vi "Create.vi"() -> (0 "error out":errorcluster, 2 "Self Event":refnum<data-value>)   [LabVIEW 2021, in "jettl.lvlib" / "Self Event.lvlib"]
uses:
  Self Event.lvlib
  Msg Strategy/Msg Strategy.lvclass
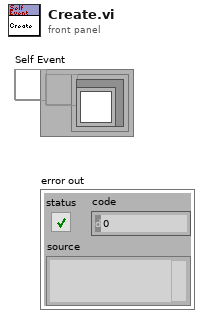
[diagram p1: front panel]
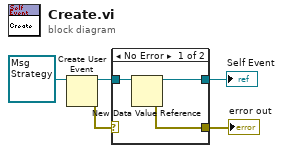
[diagram p0: block diagram]
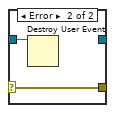
[diagram p2: hidden frame]
diagram:
  n1 = Create User Event(user event datatype=refnum<class "Msg Strategy.lvclass"> refnum ("Msg.lvclass")) -> (user event=w3:refnum<user-event>, error out=w2:errorcluster)  [unwired: 1 in]
  n2 = case shown="No Error" w2 {
    selector: w2 -> [_ w9]
    tunnel: w3 -> [w8 w10]
    tunnel: [w7 _] -> w1
    tunnel: [w6 w9] -> w5
    frame No Error {
      n3 = New Data Value Reference(data value=w8) -> (data value reference=w7:refnum<data-value>, error out=w6:errorcluster)  [unwired: 1 in]
    }
    frame Error {
      n4 = Destroy User Event(user event=w10) -> ()  [unwired: 1 in, 1 out]
    }
  }
  "error out" <- w5
  "Self Event" <- w1
